vi "run simulation.vi"(8 "error in (no error)":errorcluster, 9 "Controller Selection":T1=enum."PID", 10 "Config Path":path, 11 "Dynamic-System in":refnum<class "Dynamic-System.lvclass">) -> (0 "error out":errorcluster, 2 "XY Plot":cluster{"Time":dbl[], "Reference":dbl[]}[](graph), 3 "Dynamic-System out":refnum<class "Dynamic-System.lvclass">)   [LabVIEW 2025, in "Dynamic-System.lvclass"]
uses:
  Dynamic-System.lvclass
  controller selection.ctl
  Dynamic-System.lvclass/Dynamic-System.ctl
panel:
  in  "stop":bool
  out "Input":dbl(graph)
  out "Simulation Progress":u8(slide) scale=0.0..100.0
  out "% Complete":u8 format="%.0f%"
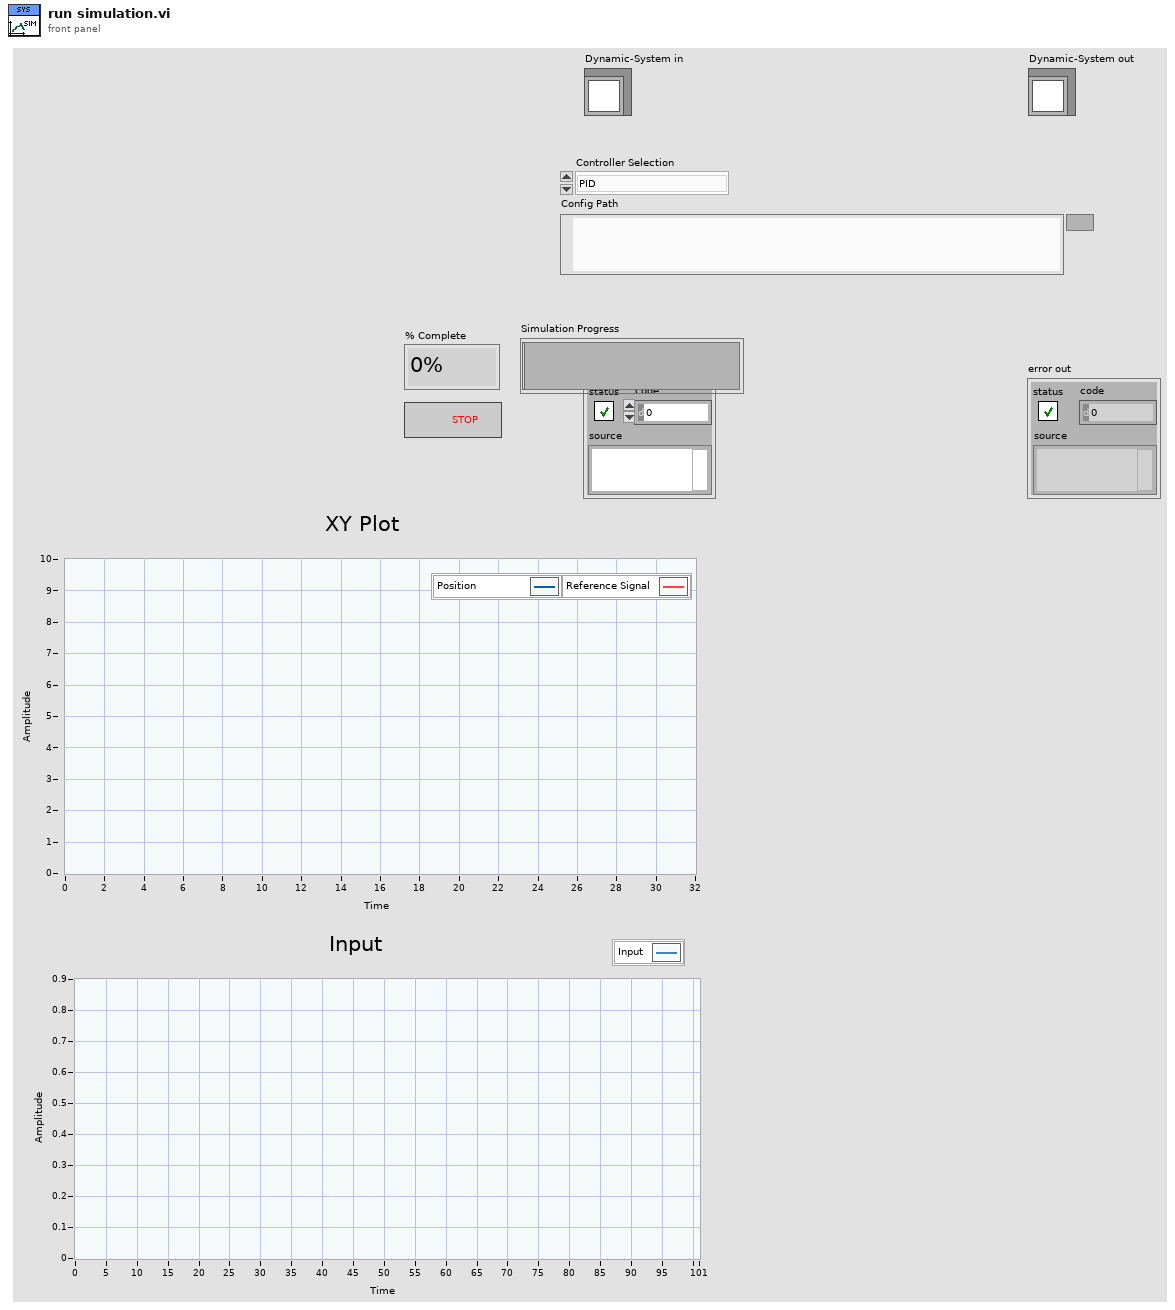
[diagram p1: front panel]
types:
  T1 = typedef "controller selection.ctl" = enum16{"No Control", "PID", "On Off"}
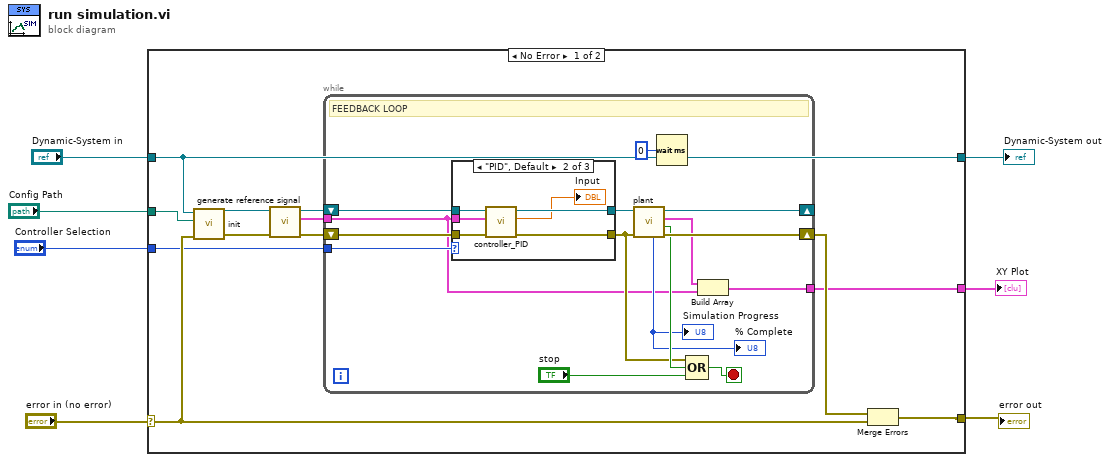
[diagram p0: block diagram]
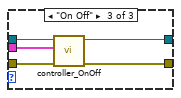
[diagram p3: hidden frame]
diagram:
  n1 = case shown="No Error" "error in (no error)" {
    selector: "error in (no error)" -> [w13 w49]
    tunnel: [w12 w49] -> w6
    tunnel: [w14 w48] -> w4
    tunnel: "Dynamic-System in" -> [w14 w48]
    tunnel: "Controller Selection" -> [w10 _]
    tunnel: [w9 _] -> w2
    tunnel: "Config Path" -> [w8 _]
    frame No Error {
      n2 = call-dynamic "init.vi"("error in (no error)"=w13, "Config Path"=w8, "Dynamic-System in"=w14) -> ("error out"=w18:errorcluster, "Dynamic-System out"=w19:refnum<class "Dynamic-System.lvclass">)  [unwired: 7 in]
      n3 = call-dynamic "generate reference signal.vi"("error in (no error)"=w18, "Dynamic-System in"=w19) -> ("error out"=w16:errorcluster, "Reference Array"=w15:cluster{"Time":dbl[], "Reference":dbl[]}, "Dynamic-System out"=w17:refnum<class "Dynamic-System.lvclass">)  [unwired: 7 in]
      n4 = while {
        shift-right: [w34] -> _
        shift-left: w17 -> [w31]
        shift-right: [w33] -> w11
        shift-left: w16 -> [w30]
        tunnel: w15 -> [w21]
        tunnel: w10 -> [w28]
        tunnel: [w20] -> w9
        stop <- w24 stop-if-true
        # "FEEDBACK LOOP"
        n5 = case shown="\"PID\", Default" w28 {
          tunnel: w31 -> [w36 w41 w47]
          tunnel: w30 -> [w35 w39 w46]
          tunnel: w21 -> [_ w38 w45]
          tunnel: [w36 w40 w44] -> w29
          tunnel: [w35 w42 w43] -> w25
          frame "No Control" {
          }
          frame "PID", Default {
            n6 = call-dynamic "controller_PID.vi"("error in (no error)"=w39, "Reference Array"=w38, "Dynamic-System in"=w41) -> ("error out"=w42:errorcluster, "Waveform Chart"=→"Input":dbl, "Dynamic-System out"=w40:refnum<class "Dynamic-System.lvclass">)  [unwired: 6 in]
          }
          frame "On Off" {
            n7 = call-dynamic "controller_OnOff.vi"("error in (no error)"=w46, "Reference Array"=w45, "Dynamic-System in"=w47) -> ("error out"=w43:errorcluster, "Dynamic-System out"=w44:refnum<class "Dynamic-System.lvclass">)  [unwired: 7 in]
          }
        }
        n8 = call-dynamic "plant.vi"("error in (no error)"=w25, "Dynamic-System in"=w29) -> ("error out"=w33:errorcluster, "End of Simulation?"=w26:bool, "output cluster"=w22:cluster{"Time":dbl[], "State 1":dbl[]}, "Dynamic-System out"=w34:refnum<class "Dynamic-System.lvclass">, "% Complete"=→"Simulation Progress" →"% Complete":u8)  [unwired: 5 in]
        n9 = Wait (ms)(milliseconds to wait=u32 0) -> ()  [unwired: 1 out]
        n10 = Compound Arithmetic op=OR(w25, w26, "stop") -> (w24:bool)
        n11 = Build Array(w22, w21) -> (w20:cluster{"Time":dbl[], "Reference":dbl[]}[])
      }
      n12 = Merge Errors(w11, w13) -> (w12:errorcluster)
    }
    frame Error {
    }
  }
  "error out" <- w6
  "Dynamic-System out" <- w4
  "XY Plot" <- w2
